vi "Update System State.vi"(0 "State Indicator":refnum<user-event>, 5 "system state message":string, 7 "additional string in":string, 11 "error in":errorcluster) -> (15 "error out":errorcluster)   [LabVIEW 2015, in "TLB` Template.lvlib"]
doc: "Update current system state.\n\n<B>Input Parameters</B>\n\n<B>system state in</B> system state control reference.\n\n<B>system state message</B> is the current system state.\n\n<B>additional string in</B> add additional text to the root state option.\n\n<B>error in</B> describes error conditions that occur before this node runs. This input provides standard error in functionality. \n\n<B>Output Parameters</B>\n\n<B>error out</B> contains error information. This output provides standard error out functionality."
uses:
  TLB` Template.lvlib
  <vilib>/regexp/Match Regular Expression.xnode
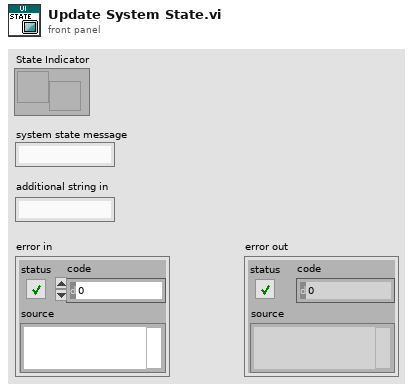
[diagram p1: front panel]
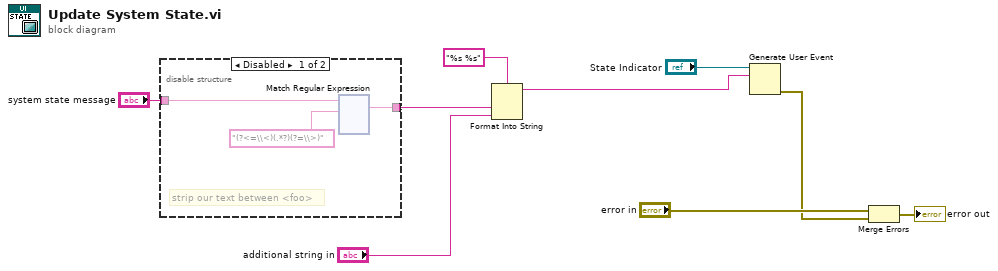
[diagram p0: block diagram]
diagram:
  n1 = disable-structure shown="Disabled" {
    disable-tunnel: "system state message" -> [w12 w127]
    disable-tunnel: [w11 w127] -> w3
    frame Disabled {
      # "strip our text between <foo>"
      n2 = xnode "Match Regular Expression"("input string"=w12, "regular expression"="(?<=\\<)(.*?)(?=\\>)") -> ("whole match"=w11:string)  [unwired: 4 in, 4 out]
    }
    frame Enabled {
    }
  }
  n3 = Format Into String(format string="%s %s", w3, "additional string in") -> (resulting string=w2:string)  [unwired: 2 in, 1 out]
  n4 = Generate User Event(user event="State Indicator", event data cluster=w2) -> (error out=w1:errorcluster)  [unwired: 2 in, 1 out]
  n5 = Merge Errors("error in", w1) -> (→"error out":errorcluster)
